vi "FITS_ReadCard.vi"(7 "Keyname":string, 8 "error in":errorcluster, 10 "ref":u64) -> (0 "error out":errorcluster, 2 "Record":string)   [LabVIEW 2016]
uses:
  usr/local/lib/libfits.so
panel:
  in  "Memory":i8[](array[numeric])
  out "result":i32
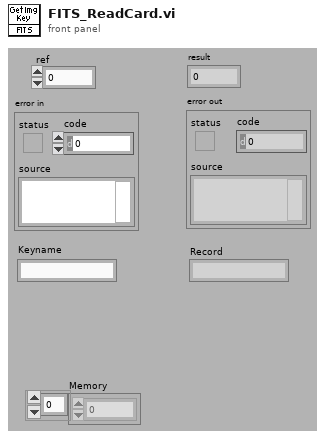
[diagram p1: front panel]
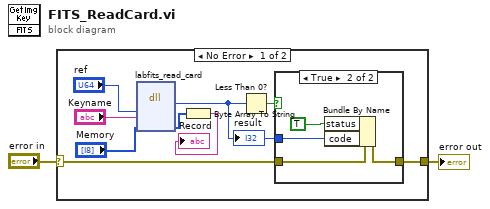
[diagram p0: block diagram]
diagram:
  n1 = case shown="No Error" "error in" {
    selector: "error in" -> [w10 w17]
    tunnel: [w9 w17] -> w1
    frame No Error {
      n2 = dll-call lib="usr/local/lib/libfits.so" fn="labfits_read_card"("ref"="ref", "keyname"="Keyname", "bufData"="Memory") -> ("return type"=w8:i32, "bufData"=w4:i8[])  [unwired: 5 in, 2 out]
      "result" <- w8
      n3 = Byte Array To String(unsigned byte array=w4) -> (string=→"Record":string)
      n4 = Less Than 0?(x=w8) -> (x < 0?=w11:bool)
      n5 = case shown="True" w11 {
        tunnel: w10 -> [w12 w14]
        tunnel: [w12 w13] -> w9
        tunnel: w8 -> [_ w15]
        frame False {
        }
        frame True {
          n6 = Bundle By Name(cluster=w14, "status"=TRUE, "code"=w15) -> (w13:errorcluster)
        }
      }
    }
    frame Error {
    }
  }
  "error out" <- w1
